vi "CLI Arguments--constant.vi"() -> (3 "Arguments":T1[](array[typedef]))   [LabVIEW 2025]
doc: "This constant contains arguments for the cli."
uses:
  <vilib>/Wiresmith Technology/G CLI/Argument Parser/Option Class/Option Configuration.ctl
  <vilib>/Wiresmith Technology/G CLI/Argument Parser/Option Class/Argument Type.ctl
  <vilib>/Wiresmith Technology/G CLI/Argument Parser/Option Class/Option.lvclass
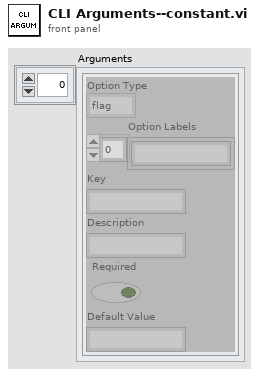
[diagram p1: front panel]
types:
  T1 = typedef "Option Parser.lvlib/Option.lvclass/Option Configuration.ctl" = cluster{"Option Type":T2, "Option Labels":string[], "Key":string, "Description":string, "Required":bool, "Default Value":string}
  T2 = typedef "Option Parser.lvlib/Option.lvclass/Argument Type.ctl" = enum16{"flag", "value"}
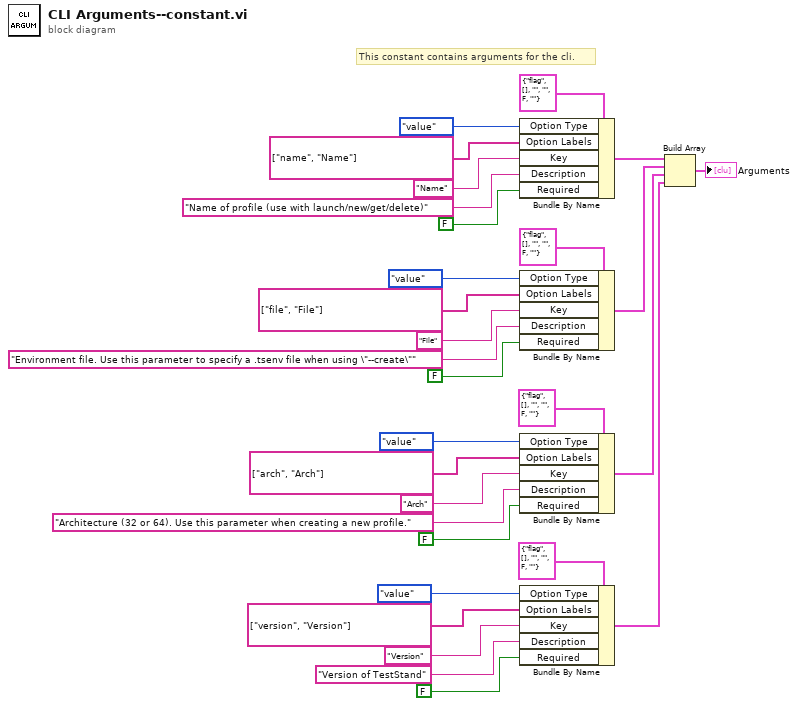
[diagram p0: block diagram]
diagram:
  # "This constant contains arguments for the cli."
  n1 = Bundle By Name(cluster=T1 {"Option Type"=enum."flag", "Option Labels"=[], "Key"="", "Description"="", "Required"=FALSE, "Default Value"=""} ("Options"), "Option Type"=Argument_Type."value", "Option Labels"=string[] ["name", "Name"], "Key"="Name", "Description"="Name of profile (use with launch/new/get/delete)", "Required"=FALSE) -> (w10:T1)
  n2 = Bundle By Name(cluster=T1 {"Option Type"=enum."flag", "Option Labels"=[], "Key"="", "Description"="", "Required"=FALSE, "Default Value"=""} ("Options"), "Option Type"=Argument_Type."value", "Option Labels"=string[] ["file", "File"], "Key"="File", "Description"="Environment file. Use this parameter to specify a .tsenv file when using \"--create\"", "Required"=FALSE) -> (w9:T1)
  n3 = Bundle By Name(cluster=T1 {"Option Type"=enum."flag", "Option Labels"=[], "Key"="", "Description"="", "Required"=FALSE, "Default Value"=""} ("Options"), "Option Type"=Argument_Type."value", "Option Labels"=string[] ["arch", "Arch"], "Key"="Arch", "Description"="Architecture (32 or 64). Use this parameter when creating a new profile.", "Required"=FALSE) -> (w8:T1)
  n4 = Bundle By Name(cluster=T1 {"Option Type"=enum."flag", "Option Labels"=[], "Key"="", "Description"="", "Required"=FALSE, "Default Value"=""} ("Options"), "Option Type"=Argument_Type."value", "Option Labels"=string[] ["version", "Version"], "Key"="Version", "Description"="Version of TestStand", "Required"=FALSE) -> (w1:T1)
  n5 = Build Array(w10, w9, w8, w1) -> (→"Arguments":T1[])
